vi "Read SFTP.vi"(8 "Error In":errorcluster, 11 "SFTP Directory In":refnum<class "SFTP Directory.lvclass">) -> (0 "Error Out":errorcluster, 2 "SFTP":refnum<class "SFTP.lvclass">, 3 "SFTP Directory Out":refnum<class "SFTP Directory.lvclass">)   [LabVIEW 2018, in "Toolkit.lvlib" / "SFTP Directory.lvclass"]
uses:
  SFTP Directory.lvclass
  SFTP/SFTP.lvclass
  SFTP Directory.lvclass/SFTP Directory.ctl
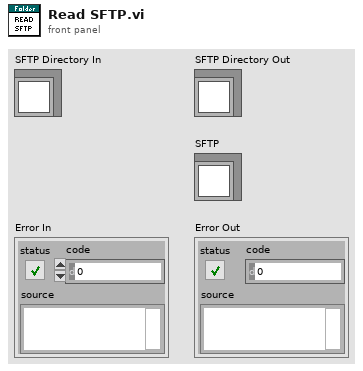
[diagram p1: front panel]
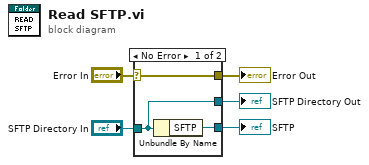
[diagram p0: block diagram]
diagram:
  n1 = case shown="No Error" "Error In" {
    selector: "Error In" -> [w8 w10]
    tunnel: "SFTP Directory In" -> [w7 w9]
    tunnel: [w7 w9] -> w3
    tunnel: [w8 w10] -> w2
    tunnel: [w6 _] -> w1
    frame No Error {
      n2 = Unbundle By Name(w7) -> ("SFTP"=w6:refnum<class "SFTP.lvclass">)
    }
    frame Error {
    }
  }
  "SFTP Directory Out" <- w3
  "Error Out" <- w2
  "SFTP" <- w1
